vi "top_display_externals.vi"(7 "AcroPDF":refnum<k7>(container), 8 "error in (no error)":errorcluster, 10 "Dynamic data":T1, 11 "Input parameters":T2={"Measurement type"=enum."Debug", "Sensor type"=enum."HPK_8in_271ch", "Identifier"="test.txt", "Open after execution?"=FALSE, "Plot after execution?"=FALSE, "Display channel"=0, "Voltage Delay (s)"=0.5, "Switch Delay (s)"=0.01, "VISA resource name source"="", "VISA resource name DMM"="", "VISA resource name LCR"="", "Compliance  Level (A)"=10.0, "Voltage Limit (V)"=1000.0, "Data storage location"="", "Scan voltages"="", "Use source as DMM?"=FALSE, "LCR signal frequenzy (Hz)"=10.0, "DMM device"=enum."Keithley2001", "Sampling number"=1, "Use env. sensors on"=enum."Sensirion sht1x/7x", "Switchboard Handle"=0, "Use Switchboard"=FALSE, "LCR signal voltage (V)"=10000.0, "Repeat"=1, "Scan voltages IV"="", "Scan voltages CV"="", "Hex pad numbers?"=FALSE, "Set measurement type"=enum."Debug", "Custom pad scan"="", "IV voltage Delay (s)"=0.5, "CV voltage Delay (s)"=0.5, "Needle measurement?"=FALSE, "Comments"="test.txt", "LCR signal frequenzy (kHz)"=10.0, "Compliance  Level (uA)"=10.0, "Open Correction Array"=array2304x3[6912 elements], "Current set voltage"=0.0, "Last set voltage"=0.0, "Current channel"=0, "Last OpenCorrection index"=-1, "Total curr/vltg every x steps"=10, "Current channel iteration"=0, "No CV corrections"=FALSE, "Mapfile"="", "Corrfile"="", "IV voltage file"=path "", "CV voltage file"=path "", "IV Switch Delay (s)"=0.01, "CV Switch Delay (s)"=0.01, "Invert polarity"=FALSE, "Set debug dirs"=FALSE, "Is n on p"=FALSE, "Source interlock?"=TRUE, "Voltage file used?"=FALSE, "Pad mask"="", "Mask pad above (uA)"=1.0, "LCR device"=enum."LCR_E4980", "Source device"=enum."Source_2410", "HexPlot binary path"="", "PadReductionFactor"=1.0, "Temperature degC"="", "Fluence [neq]"="", "Annealing [min]"=""} {"CV Switch Delay (s)" format="%#_13g"; "IV Switch Delay (s)" format="%#_13g"; "Last set voltage" format="%#_13g"; "Current set voltage" format="%#_13g"; "CV voltage Delay (s)" format="%#_13g"; "IV voltage Delay (s)" format="%#_13g"; "Voltage Limit (V)" format="%#_13g"; "Voltage Delay (s)" format="%#_13g"; "Switch Delay (s)" format="%#_13g"}) -> (0 "error out":errorcluster, 2 "Dynamic data":T1, 3 "Input parameters":T2={"Measurement type"=enum."Debug", "Sensor type"=enum."HPK_8in_271ch", "Identifier"="test.txt", "Open after execution?"=FALSE, "Plot after execution?"=FALSE, "Display channel"=0, "Voltage Delay (s)"=0.5, "Switch Delay (s)"=0.01, "VISA resource name source"="", "VISA resource name DMM"="", "VISA resource name LCR"="", "Compliance  Level (A)"=10.0, "Voltage Limit (V)"=1000.0, "Data storage location"="", "Scan voltages"="", "Use source as DMM?"=FALSE, "LCR signal frequenzy (Hz)"=10.0, "DMM device"=enum."Keithley2001", "Sampling number"=1, "Use env. sensors on"=enum."Sensirion sht1x/7x", "Switchboard Handle"=0, "Use Switchboard"=FALSE, "LCR signal voltage (V)"=10000.0, "Repeat"=1, "Scan voltages IV"="", "Scan voltages CV"="", "Hex pad numbers?"=FALSE, "Set measurement type"=enum."Debug", "Custom pad scan"="", "IV voltage Delay (s)"=0.5, "CV voltage Delay (s)"=0.5, "Needle measurement?"=FALSE, "Comments"="test.txt", "LCR signal frequenzy (kHz)"=10.0, "Compliance  Level (uA)"=10.0, "Open Correction Array"=array2304x3[6912 elements], "Current set voltage"=0.0, "Last set voltage"=0.0, "Current channel"=0, "Last OpenCorrection index"=-1, "Total curr/vltg every x steps"=10, "Current channel iteration"=0, "No CV corrections"=FALSE, "Mapfile"="", "Corrfile"="", "IV voltage file"=path "", "CV voltage file"=path "", "IV Switch Delay (s)"=0.01, "CV Switch Delay (s)"=0.01, "Invert polarity"=FALSE, "Set debug dirs"=FALSE, "Is n on p"=FALSE, "Source interlock?"=TRUE, "Voltage file used?"=FALSE, "Pad mask"="", "Mask pad above (uA)"=1.0, "LCR device"=enum."LCR_E4980", "Source device"=enum."Source_2410", "HexPlot binary path"="", "PadReductionFactor"=1.0, "Temperature degC"="", "Fluence [neq]"="", "Annealing [min]"=""} {"CV Switch Delay (s)" format="%#_13g"; "IV Switch Delay (s)" format="%#_13g"; "Last set voltage" format="%#_13g"; "Current set voltage" format="%#_13g"; "CV voltage Delay (s)" format="%#_13g"; "IV voltage Delay (s)" format="%#_13g"; "Voltage Limit (V)" format="%#_13g"; "Voltage Delay (s)" format="%#_13g"; "Switch Delay (s)" format="%#_13g"})   [LabVIEW 2020]
doc: "Handles the PDF display."
uses:
  input_params.ctl
  data_dynamic.ctl
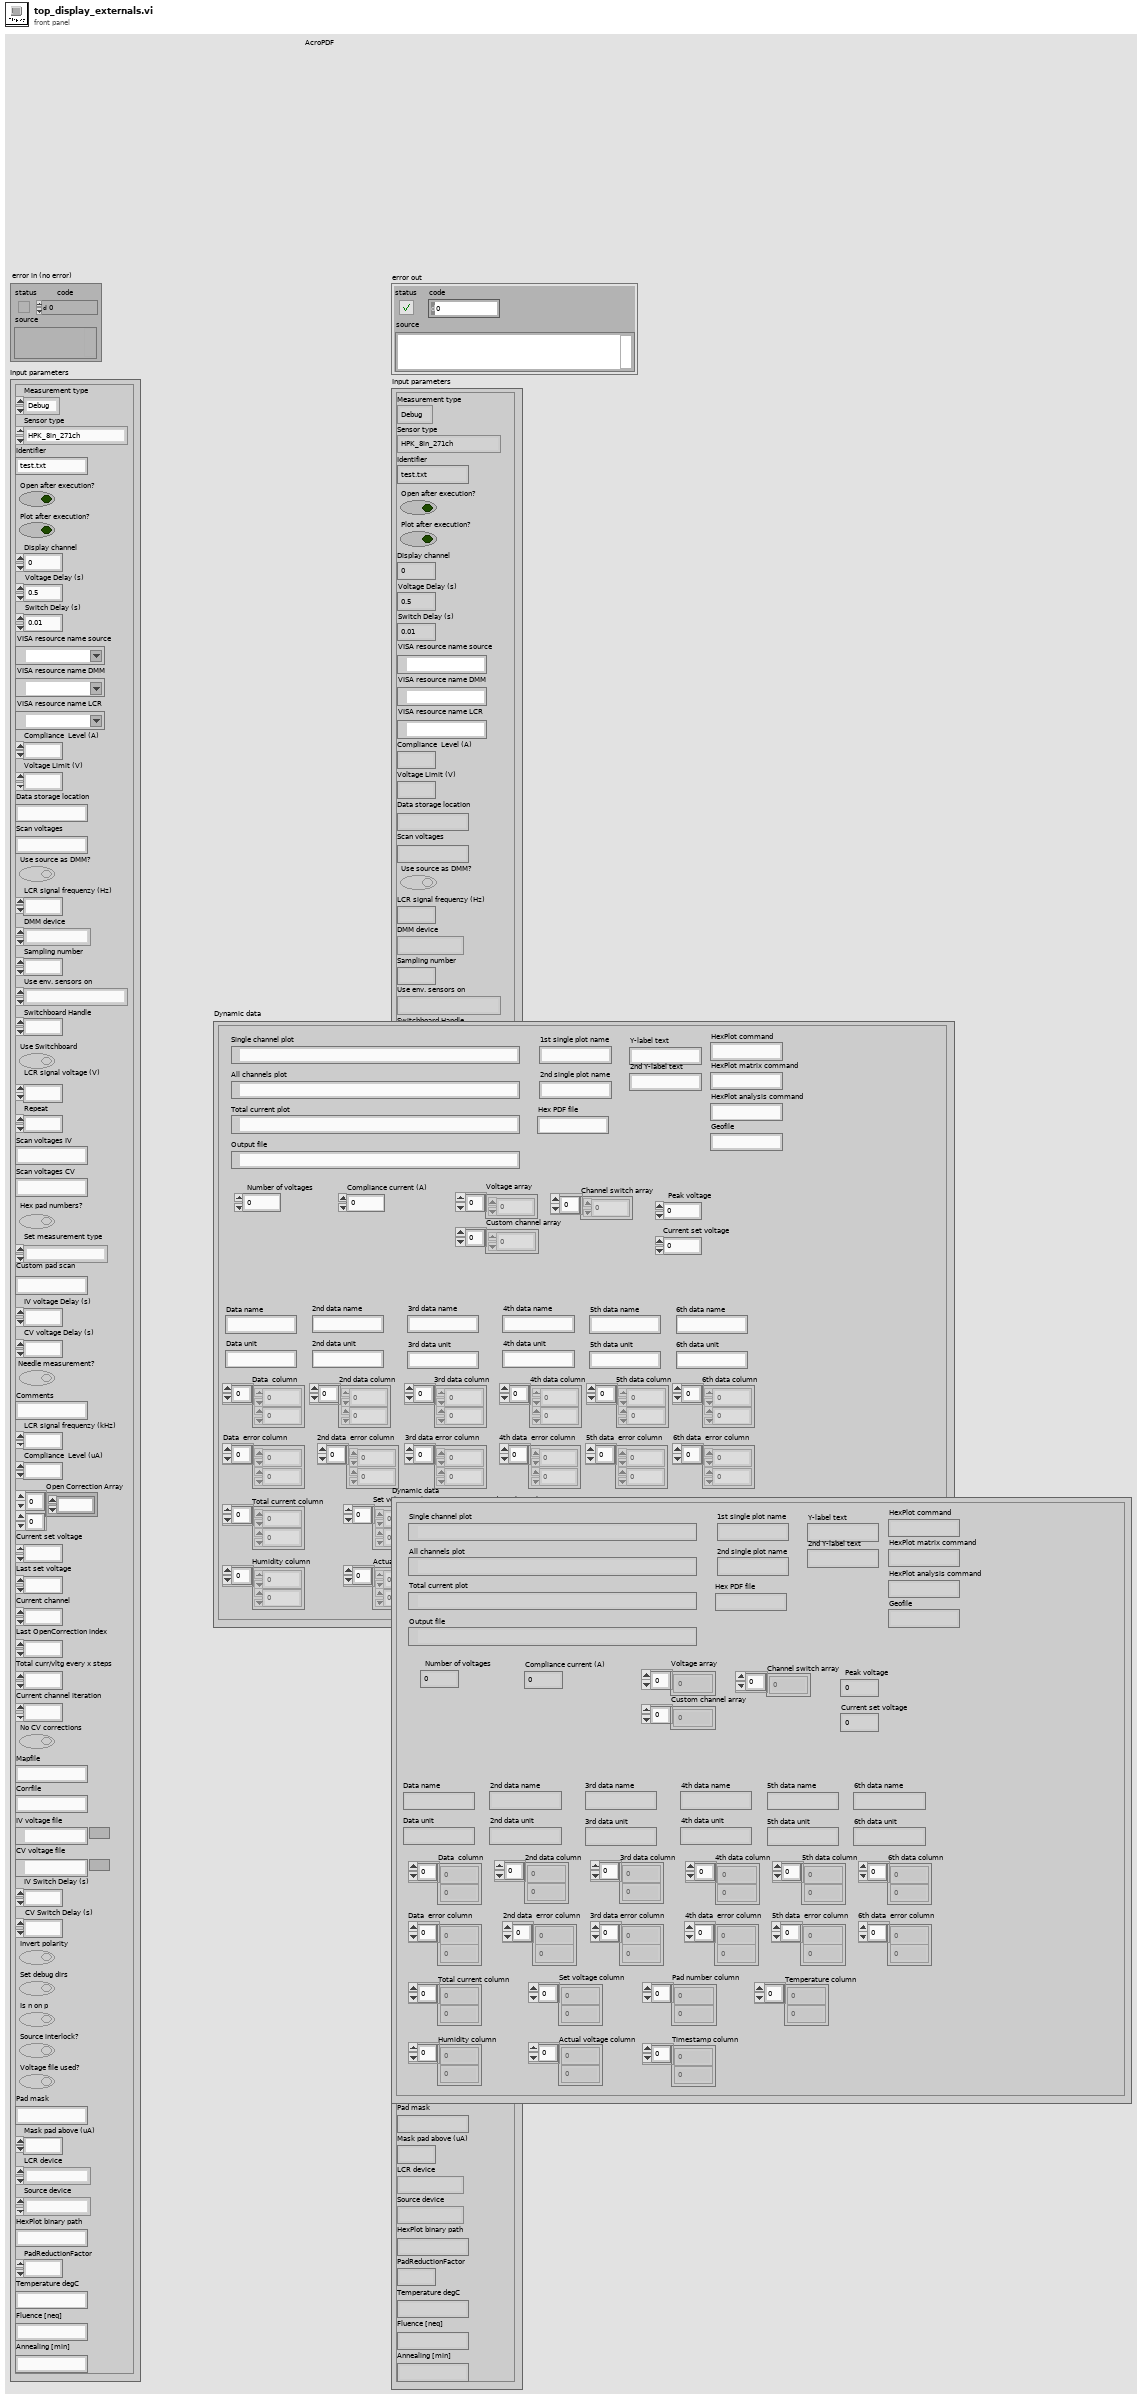
[diagram p1: front panel]
types:
  T1 = typedef "data_dynamic.ctl" = cluster{"Output file":path, "Y-label text":string, "Current set voltage":dbl, "Set voltage column":dbl[], "Pad number column":dbl[], "Data  column":dbl[], "Number of voltages":i32, "Compliance current (A)":dbl, "Geofile":string, "Peak voltage":dbl, "Hex PDF file":string, "Voltage array":dbl[], "Total current column":dbl[], "Timestamp column":dbl[], "Data name":string, "Data unit":string, "2nd data column":dbl[], "2nd data name":string, "2nd data unit":string, "3rd data column":dbl[], "4th data column":dbl[], "3rd data name":string, "3rd data unit":string, "4th data name":string, "4th data unit":string, "Actual voltage column":dbl[], "2nd Y-label text":string, "Single channel plot":path, "Temperature column":dbl[], "Humidity column":dbl[], "Channel switch array":i32[], "1st single plot name":string, "2nd single plot name":string, "All channels plot":path, "HexPlot command":string, "Custom channel array":i32[], "Data  error column":dbl[], "2nd data  error column":dbl[], "3rd data error column":dbl[], "4th data  error column":dbl[], "Total current plot":path, "5th data column":dbl[], "5th data  error column":dbl[], "6th data column":dbl[], "6th data  error column":dbl[], "5th data name":string, "5th data unit":string, "6th data name":string, "6th data unit":string, "HexPlot matrix command":string, "HexPlot analysis command":string}
  T2 = typedef "input_params.ctl" = cluster{"Measurement type":enum16{"IV", "CV", "Debug", "Test_contact"}, "Sensor type":enum16{"HPK_6in_135ch", "HPK_8in_271ch", "IFX_8in_256ch", "Diode", "HPK_6in_239ch", "Full_Matrix", "HPK_8in_271ch_full", "LumiCal", "HPK_8in_444ch", "HPK_8in_198ch_2019", "HPK_8in_MGW_LD_full", "HPK_8in_MGW_LD_a_type_top", "HPK_8in_MGW_LD_a_type_bottom", "HPK_8in_MGW_LD_b_type_left", "HPK_8in_MGW_LD_b_type_right", "HPK_8in_MGW_LD_c_type_left", "HPK_8in_MGW_LD_c_type_right", "HPK_8in_MGW_HD_full", "HPK_8in_MGW_HD_a_type_top", "HPK_8in_MGW_HD_a_type_bottom", "HPK_8in_MGW_HD_b_type_left", "HPK_8in_MGW_HD_b_type_right", "HPK_8in_MGW_HD_c_type_left", "HPK_8in_MGW_HD_c_type_right", "CALICE_6in_256ch"}, "Identifier":string, "Open after execution?":bool, "Plot after execution?":bool, "Display channel":i32, "Voltage Delay (s)":dbl, "Switch Delay (s)":dbl, "VISA resource name source":refnum<visa-resource-name>, "VISA resource name DMM":refnum<visa-resource-name>, "VISA resource name LCR":refnum<visa-resource-name>, "Compliance  Level (A)":dbl, "Voltage Limit (V)":dbl, "Data storage location":string, "Scan voltages":string, "Use source as DMM?":bool, "LCR signal frequenzy (Hz)":dbl, "DMM device":enum16{"Keithley2001", "Keithley2450", "Keithley2410", "Keithley6485", "Keithley6487", "Keithley6517"}, "Sampling number":i32, "Use env. sensors on":enum16{"Sensirion sht1x/7x", "Switch Matrix", "Probecard"}, "Switchboard Handle":u32, "Use Switchboard":bool, "LCR signal voltage (V)":dbl, "Repeat":i32, "Scan voltages IV":string, "Scan voltages CV":string, "Hex pad numbers?":bool, "Set measurement type":enum16{"IV", "CV", "Debug", "Test_contact", "IV+CV"}, "Custom pad scan":string, "IV voltage Delay (s)":dbl, "CV voltage Delay (s)":dbl, "Needle measurement?":bool, "Comments":string, "LCR signal frequenzy (kHz)":dbl, "Compliance  Level (uA)":dbl, "Open Correction Array":dbl[][], "Current set voltage":dbl, "Last set voltage":dbl, "Current channel":i32, "Last OpenCorrection index":i32, "Total curr/vltg every x steps":i32, "Current channel iteration":i32, "No CV corrections":bool, "Mapfile":string, "Corrfile":string, "IV voltage file":path, "CV voltage file":path, "IV Switch Delay (s)":dbl, "CV Switch Delay (s)":dbl, "Invert polarity":bool, "Set debug dirs":bool, "Is n on p":bool, "Source interlock?":bool, "Voltage file used?":bool, "Pad mask":string, "Mask pad above (uA)":dbl, "LCR device":enum16{"LCR_E4980", "AGILENT_4263X"}, "Source device":enum16{"Source_2410", "Source_6487"}, "HexPlot binary path":string, "PadReductionFactor":dbl, "Temperature degC":string, "Fluence [neq]":string, "Annealing [min]":string}
  T3 = enum16{"HPK_6in_135ch", "HPK_8in_271ch", "IFX_8in_256ch", "Diode", "HPK_6in_239ch", "Full_Matrix", "HPK_8in_271ch_full", "LumiCal", "HPK_8in_444ch", "HPK_8in_198ch_2019", "HPK_8in_MGW_LD_full", "HPK_8in_MGW_LD_a_type_top", "HPK_8in_MGW_LD_a_type_bottom", "HPK_8in_MGW_LD_b_type_left", "HPK_8in_MGW_LD_b_type_right", "HPK_8in_MGW_LD_c_type_left", "HPK_8in_MGW_LD_c_type_right", "HPK_8in_MGW_HD_full", "HPK_8in_MGW_HD_a_type_top", "HPK_8in_MGW_HD_a_type_bottom", "HPK_8in_MGW_HD_b_type_left", "HPK_8in_MGW_HD_b_type_right", "HPK_8in_MGW_HD_c_type_left", "HPK_8in_MGW_HD_c_type_right", "CALICE_6in_256ch"}
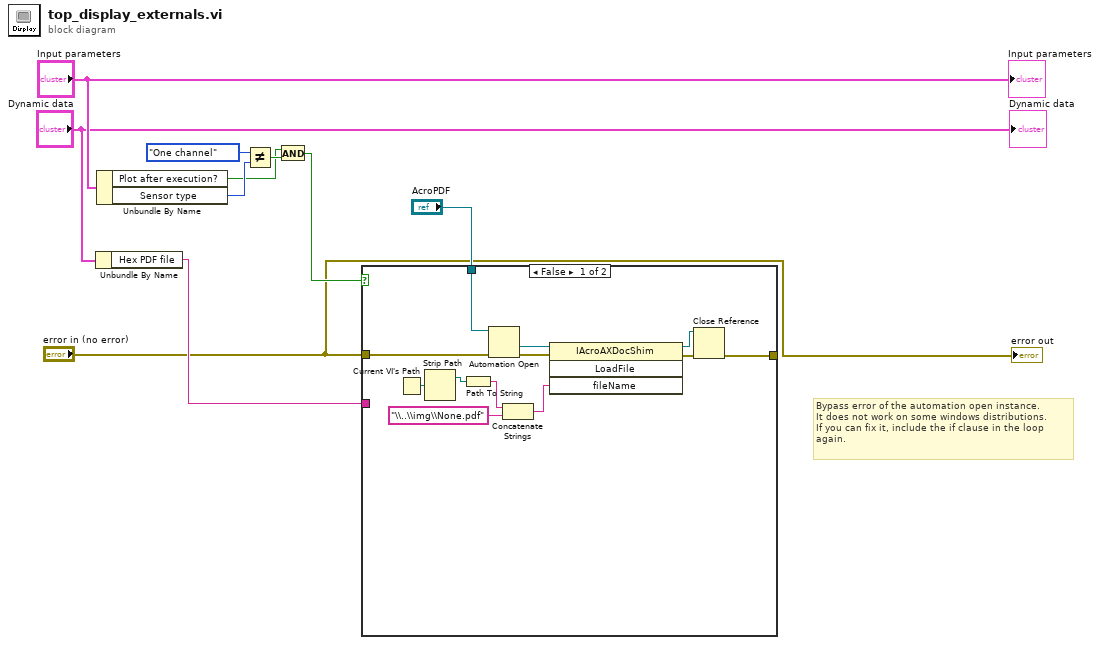
[diagram p0: block diagram]
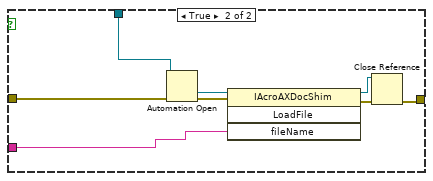
[diagram p2: hidden frame]
diagram:
  # "Bypass error of the automation open instance. \nIt does not work on some windows distributions.\nIf you can fix it, include the if clause in the loop\nagain."
  n1 = Unbundle By Name("Dynamic data") -> ("Hex PDF file"=w8:string)
  n2 = Unbundle By Name("Input parameters") -> ("Plot after execution?"=w4:bool, "Sensor type"=w7:T3)
  n3 = Not Equal?(x=enum16{"6''", "8''", "One channel"}."One channel", y=w7) -> (x != y?=w5:bool)
  n4 = And(x=w4, y=w5) -> (x .and. y?=w3:bool)
  n5 = case shown="False" w3 {
    tunnel: "error in (no error)" -> [w13 w24]
    tunnel: [w11 w30] -> _
    tunnel: "AcroPDF" -> [w12 w29]
    tunnel: w8 -> [_ w23]
    frame False {
      n6 = Current VI's Path() -> (path=w17:path)
      n7 = Strip Path(path=w17) -> (stripped path=w16:path)  [unwired: 1 out]
      n8 = Path To String(path=w16) -> (string=w15:string)
      n9 = Automation Open(error in (no error)=w13, Automation Refnum=w12) -> (Automation Refnum=w22:refnum<k7>, error out=w21:errorcluster)  [unwired: 2 in]
      n10 = Concatenate Strings(w15, "\\..\\img\\None.pdf" ("string")) -> (w14:string)
      n11 = invoke class="IAcroAXDocShim" method="LoadFile"(reference=w22, error in=w21, "fileName"=w14) -> (reference out=w20:refnum<k7>, error out=w19:errorcluster)  [unwired: 1 in, 2 out]
      n12 = Close Reference(reference=w20, error in (no error)=w19) -> (error out=w11:errorcluster)
    }
    frame True {
      n13 = Automation Open(error in (no error)=w24, Automation Refnum=w29) -> (Automation Refnum=w28:refnum<k7>, error out=w27:errorcluster)  [unwired: 2 in]
      n14 = invoke class="IAcroAXDocShim" method="LoadFile"(reference=w28, error in=w27, "fileName"=w23) -> (reference out=w26:refnum<k7>, error out=w25:errorcluster)  [unwired: 1 in, 2 out]
      n15 = Close Reference(reference=w26, error in (no error)=w25) -> (error out=w30:errorcluster)
    }
  }
  "error out" <- "error in (no error)"
  "Input parameters" <- "Input parameters"
  "Dynamic data" <- "Dynamic data"
